vi "Start.vi"(6 "Load FP? (T)":bool=TRUE, 8 "error in (no error)":errorcluster, 9 "Data":string, 10 "Name":string, 11 "VI Reference in":variant) -> (0 "error out":errorcluster, 2 "Generic VI Reference":refnum<vi>, 3 "VI Reference out":variant)   [LabVIEW 2021, in "Thread.lvlib"]
uses:
  Thread.lvlib
  <vilib>/Utility/error.llb/Error Cluster From Error Code.vi
  <vilib>/ErrorRing/Error Ring.xnode
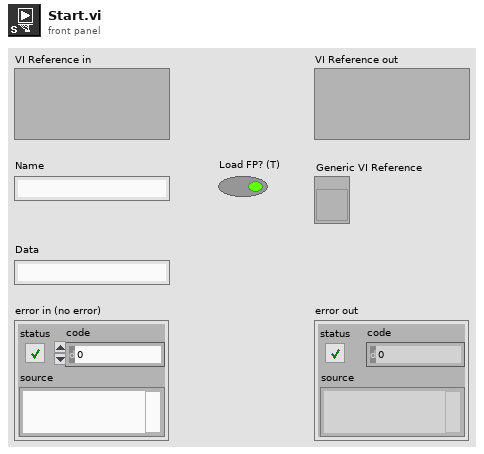
[diagram p1: front panel]
types:
  T1 = enum32{"Invalid", "Standard", "Closed", "Hidden", "Minimized", "Maximized"}
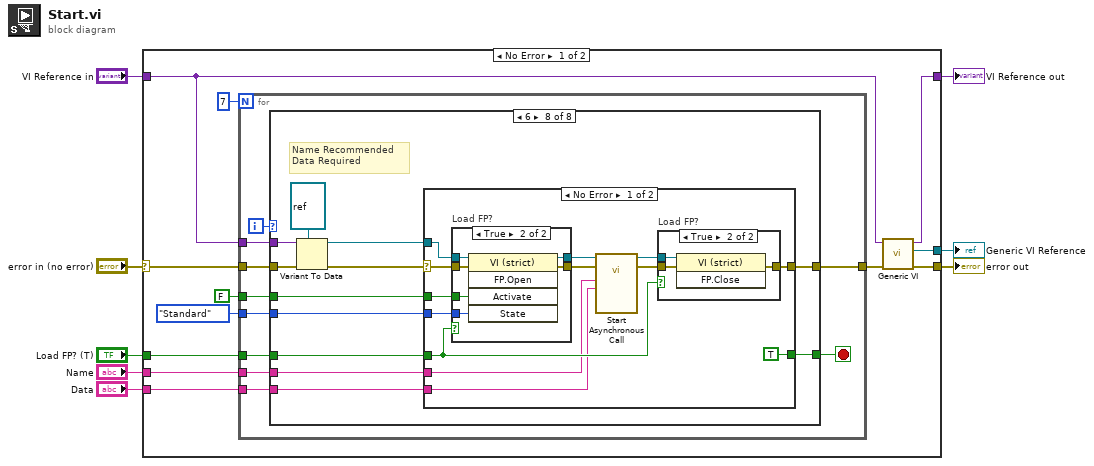
[diagram p0: block diagram]
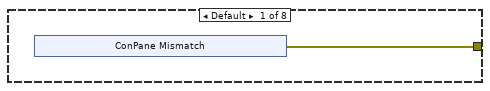
[diagram p2: hidden frame]
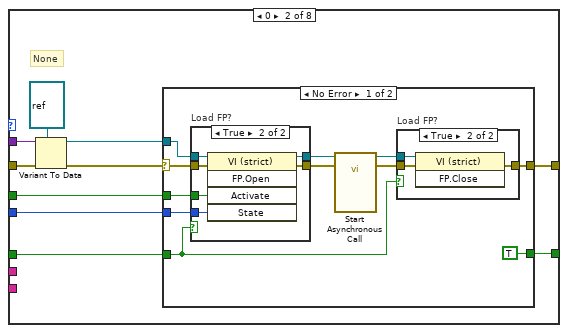
[diagram p3: hidden frame]
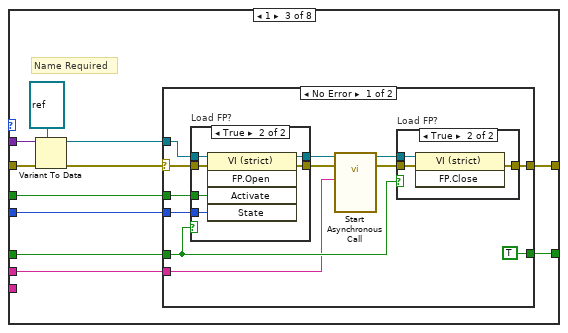
[diagram p7: hidden frame]
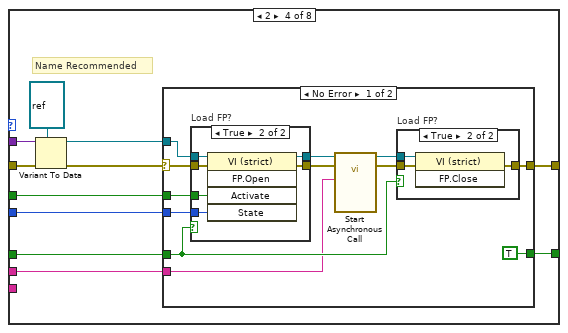
[diagram p11: hidden frame]
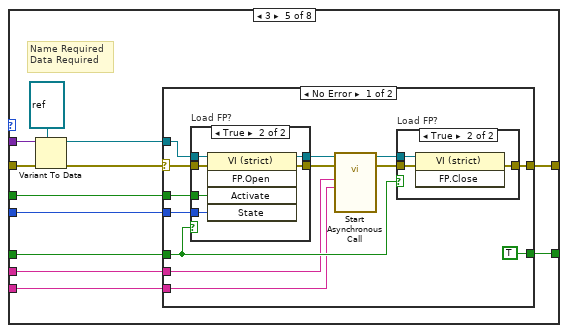
[diagram p15: hidden frame]
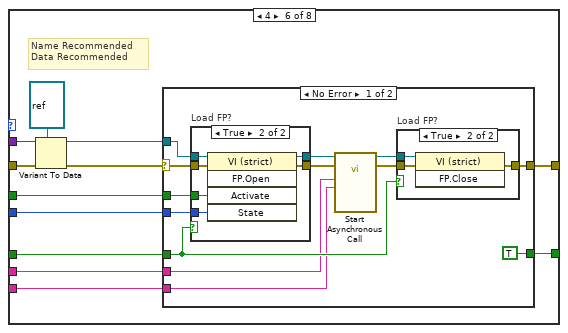
[diagram p19: hidden frame]
diagram:
  n1 = case shown="No Error" "error in (no error)" {
    selector: "error in (no error)" -> [w20 w294]
    tunnel: "VI Reference in" -> [w9 _]
    tunnel: [w12 w294] -> w7
    tunnel: [w10 _] -> w6
    tunnel: [w11 _] -> w5
    tunnel: "Load FP? (T)" -> [w18 _]
    tunnel: "Name" -> [w17 _]
    tunnel: "Data" -> [w16 _]
    frame No Error {
      n2 = for {
        N: 7 -> [_]
        tunnel: w9 -> [w29]
        tunnel: w20 -> [w30]
        tunnel: [w27] -> w13
        tunnel: w18 -> [w26]
        tunnel: w17 -> [w25]
        tunnel: w16 -> [w24]
        tunnel: FALSE ("Activate?") -> [w23]
        tunnel: T1."Standard" ("State") -> [w22]
        i -> [w28]
        stop <- w21 stop-if-true
        n3 = case shown="6" w28 {
          tunnel: w30 -> [_ w45 w80 w116 w153 w191 w229 w267]
          tunnel: w29 -> [_ w43 w78 w114 w151 w189 w227 w265]
          tunnel: [w31 w41 w76 w112 w149 w187 w225 w263] -> w27
          tunnel: w26 -> [_ w39 w75 w111 w148 w186 w224 w262]
          tunnel: w25 -> [_ _ w70 w106 w144 w182 w220 w258]
          tunnel: w24 -> [_ _ _ _ w142 w181 w219 w257]
          tunnel: w23 -> [_ w38 w74 w110 w147 w185 w223 w261]
          tunnel: w22 -> [_ w37 w73 w109 w146 w184 w222 w260]
          tunnel: [_ w36 w72 w108 w145 w183 w221 w259] -> w21
          frame Default {
            n4 = xnode "ConPane Mismatch"() -> ("error out"=w31:errorcluster)
          }
          frame 0 {
            # "None"
            n5 = Variant To Data(error in=w45, type=refnum<vi> refnum ("VI Refnum"), Variant=w43) -> (data=w42:refnum<vi>, error out=w44:errorcluster)
            n6 = case shown="No Error" w44 {
              selector: w44 -> [w56 w69]
              tunnel: w42 -> [w53 _]
              tunnel: [w51 w69] -> w41
              tunnel: w39 -> [w49 _]
              tunnel: w38 -> [w48 _]
              tunnel: w37 -> [w47 _]
              tunnel: [TRUE _] -> w36
              frame No Error {
                n7 = case "Load FP?" shown="True" w49 {
                  tunnel: w56 -> [w62 w68]
                  tunnel: [w62 w67] -> w54
                  tunnel: w53 -> [w61 w66]
                  tunnel: [w61 w65] -> w52
                  tunnel: w48 -> [_ w64]
                  tunnel: w47 -> [_ w63]
                  frame False {
                  }
                  frame True {
                    n8 = invoke class="VI (strict)" method="FP.Open"(reference=w66, error in=w68, "Activate"=w64, "State"=w63) -> (reference out=w65:refnum<vi>, error out=w67:errorcluster)  [unwired: 1 in, 3 out]
                  }
                }
                n9 = call-by-ref "Start Asynchronous Call"(reference=w52, error in=w54) -> (reference out=w50:refnum<vi>, error out=w55:errorcluster)  [unwired: 12 in]
                n10 = case "Load FP?" shown="True" w49 {
                  tunnel: w55 -> [w57 w60]
                  tunnel: [w57 w59] -> w51
                  tunnel: w50 -> [_ w58]
                  frame False {
                  }
                  frame True {
                    n11 = invoke class="VI (strict)" method="FP.Close"(reference=w58, error in=w60) -> (error out=w59:errorcluster)  [unwired: 1 in, 2 out]
                  }
                }
              }
              frame Error {
              }
            }
          }
          frame 1 {
            # "Name Required"
            n12 = Variant To Data(error in=w80, type=refnum<vi> refnum ("VI Refnum"), Variant=w78) -> (data=w77:refnum<vi>, error out=w79:errorcluster)
            n13 = case shown="No Error" w79 {
              selector: w79 -> [w92 w105]
              tunnel: w77 -> [w89 _]
              tunnel: [w87 w105] -> w76
              tunnel: w75 -> [w85 _]
              tunnel: w74 -> [w84 _]
              tunnel: w73 -> [w83 _]
              tunnel: [TRUE _] -> w72
              tunnel: w70 -> [w81 _]
              frame No Error {
                n14 = case "Load FP?" shown="True" w85 {
                  tunnel: w92 -> [w98 w104]
                  tunnel: [w98 w103] -> w90
                  tunnel: w89 -> [w97 w102]
                  tunnel: [w97 w101] -> w88
                  tunnel: w84 -> [_ w100]
                  tunnel: w83 -> [_ w99]
                  frame False {
                  }
                  frame True {
                    n15 = invoke class="VI (strict)" method="FP.Open"(reference=w102, error in=w104, "Activate"=w100, "State"=w99) -> (reference out=w101:refnum<vi>, error out=w103:errorcluster)  [unwired: 1 in, 3 out]
                  }
                }
                n16 = call-by-ref "Start Asynchronous Call"(reference=w88, error in=w90, "Name"=w81) -> (reference out=w86:refnum<vi>, error out=w91:errorcluster)  [unwired: 11 in]
                n17 = case "Load FP?" shown="True" w85 {
                  tunnel: w91 -> [w93 w96]
                  tunnel: [w93 w95] -> w87
                  tunnel: w86 -> [_ w94]
                  frame False {
                  }
                  frame True {
                    n18 = invoke class="VI (strict)" method="FP.Close"(reference=w94, error in=w96) -> (error out=w95:errorcluster)  [unwired: 1 in, 2 out]
                  }
                }
              }
              frame Error {
              }
            }
          }
          frame 2 {
            # "Name Recommended"
            n19 = Variant To Data(error in=w116, type=refnum<vi> refnum ("VI Refnum"), Variant=w114) -> (data=w113:refnum<vi>, error out=w115:errorcluster)
            n20 = case shown="No Error" w115 {
              selector: w115 -> [w128 w141]
              tunnel: w113 -> [w125 _]
              tunnel: [w123 w141] -> w112
              tunnel: w111 -> [w121 _]
              tunnel: w110 -> [w120 _]
              tunnel: w109 -> [w119 _]
              tunnel: [TRUE _] -> w108
              tunnel: w106 -> [w117 _]
              frame No Error {
                n21 = case "Load FP?" shown="True" w121 {
                  tunnel: w128 -> [w134 w140]
                  tunnel: [w134 w139] -> w126
                  tunnel: w125 -> [w133 w138]
                  tunnel: [w133 w137] -> w124
                  tunnel: w120 -> [_ w136]
                  tunnel: w119 -> [_ w135]
                  frame False {
                  }
                  frame True {
                    n22 = invoke class="VI (strict)" method="FP.Open"(reference=w138, error in=w140, "Activate"=w136, "State"=w135) -> (reference out=w137:refnum<vi>, error out=w139:errorcluster)  [unwired: 1 in, 3 out]
                  }
                }
                n23 = call-by-ref "Start Asynchronous Call"(reference=w124, error in=w126, "Name"=w117) -> (reference out=w122:refnum<vi>, error out=w127:errorcluster)  [unwired: 11 in]
                n24 = case "Load FP?" shown="True" w121 {
                  tunnel: w127 -> [w129 w132]
                  tunnel: [w129 w131] -> w123
                  tunnel: w122 -> [_ w130]
                  frame False {
                  }
                  frame True {
                    n25 = invoke class="VI (strict)" method="FP.Close"(reference=w130, error in=w132) -> (error out=w131:errorcluster)  [unwired: 1 in, 2 out]
                  }
                }
              }
              frame Error {
              }
            }
          }
          frame 3 {
            # "Name Required\nData Required"
            n26 = Variant To Data(error in=w153, type=refnum<vi> refnum ("VI Refnum"), Variant=w151) -> (data=w150:refnum<vi>, error out=w152:errorcluster)
            n27 = case shown="No Error" w152 {
              selector: w152 -> [w166 w179]
              tunnel: w150 -> [w163 _]
              tunnel: [w161 w179] -> w149
              tunnel: w148 -> [w159 _]
              tunnel: w147 -> [w158 _]
              tunnel: w146 -> [w157 _]
              tunnel: [TRUE _] -> w145
              tunnel: w144 -> [w155 _]
              tunnel: w142 -> [w154 _]
              frame No Error {
                n28 = case "Load FP?" shown="True" w159 {
                  tunnel: w166 -> [w172 w178]
                  tunnel: [w172 w177] -> w164
                  tunnel: w163 -> [w171 w176]
                  tunnel: [w171 w175] -> w162
                  tunnel: w158 -> [_ w174]
                  tunnel: w157 -> [_ w173]
                  frame False {
                  }
                  frame True {
                    n29 = invoke class="VI (strict)" method="FP.Open"(reference=w176, error in=w178, "Activate"=w174, "State"=w173) -> (reference out=w175:refnum<vi>, error out=w177:errorcluster)  [unwired: 1 in, 3 out]
                  }
                }
                n30 = call-by-ref "Start Asynchronous Call"(reference=w162, error in=w164, "Data"=w154, "Name"=w155) -> (reference out=w160:refnum<vi>, error out=w165:errorcluster)  [unwired: 10 in]
                n31 = case "Load FP?" shown="True" w159 {
                  tunnel: w165 -> [w167 w170]
                  tunnel: [w167 w169] -> w161
                  tunnel: w160 -> [_ w168]
                  frame False {
                  }
                  frame True {
                    n32 = invoke class="VI (strict)" method="FP.Close"(reference=w168, error in=w170) -> (error out=w169:errorcluster)  [unwired: 1 in, 2 out]
                  }
                }
              }
              frame Error {
              }
            }
          }
          frame 4 {
            # "Name Recommended\nData Recommended"
            n33 = Variant To Data(error in=w191, type=refnum<vi> refnum ("VI Refnum"), Variant=w189) -> (data=w188:refnum<vi>, error out=w190:errorcluster)
            n34 = case shown="No Error" w190 {
              selector: w190 -> [w204 w217]
              tunnel: w188 -> [w201 _]
              tunnel: [w199 w217] -> w187
              tunnel: w186 -> [w197 _]
              tunnel: w185 -> [w196 _]
              tunnel: w184 -> [w195 _]
              tunnel: [TRUE _] -> w183
              tunnel: w182 -> [w193 _]
              tunnel: w181 -> [w192 _]
              frame No Error {
                n35 = case "Load FP?" shown="True" w197 {
                  tunnel: w204 -> [w210 w216]
                  tunnel: [w210 w215] -> w202
                  tunnel: w201 -> [w209 w214]
                  tunnel: [w209 w213] -> w200
                  tunnel: w196 -> [_ w212]
                  tunnel: w195 -> [_ w211]
                  frame False {
                  }
                  frame True {
                    n36 = invoke class="VI (strict)" method="FP.Open"(reference=w214, error in=w216, "Activate"=w212, "State"=w211) -> (reference out=w213:refnum<vi>, error out=w215:errorcluster)  [unwired: 1 in, 3 out]
                  }
                }
                n37 = call-by-ref "Start Asynchronous Call"(reference=w200, error in=w202, "Data"=w192, "Name"=w193) -> (reference out=w198:refnum<vi>, error out=w203:errorcluster)  [unwired: 10 in]
                n38 = case "Load FP?" shown="True" w197 {
                  tunnel: w203 -> [w205 w208]
                  tunnel: [w205 w207] -> w199
                  tunnel: w198 -> [_ w206]
                  frame False {
                  }
                  frame True {
                    n39 = invoke class="VI (strict)" method="FP.Close"(reference=w206, error in=w208) -> (error out=w207:errorcluster)  [unwired: 1 in, 2 out]
                  }
                }
              }
              frame Error {
              }
            }
          }
          frame 5 {
            # "Name Required\nData Recommended"
            n40 = Variant To Data(error in=w229, type=refnum<vi> refnum ("VI Refnum"), Variant=w227) -> (data=w226:refnum<vi>, error out=w228:errorcluster)
            n41 = case shown="No Error" w228 {
              selector: w228 -> [w242 w255]
              tunnel: w226 -> [w239 _]
              tunnel: [w237 w255] -> w225
              tunnel: w224 -> [w235 _]
              tunnel: w223 -> [w234 _]
              tunnel: w222 -> [w233 _]
              tunnel: [TRUE _] -> w221
              tunnel: w220 -> [w231 _]
              tunnel: w219 -> [w230 _]
              frame No Error {
                n42 = case "Load FP?" shown="True" w235 {
                  tunnel: w242 -> [w248 w254]
                  tunnel: [w248 w253] -> w240
                  tunnel: w239 -> [w247 w252]
                  tunnel: [w247 w251] -> w238
                  tunnel: w234 -> [_ w250]
                  tunnel: w233 -> [_ w249]
                  frame False {
                  }
                  frame True {
                    n43 = invoke class="VI (strict)" method="FP.Open"(reference=w252, error in=w254, "Activate"=w250, "State"=w249) -> (reference out=w251:refnum<vi>, error out=w253:errorcluster)  [unwired: 1 in, 3 out]
                  }
                }
                n44 = call-by-ref "Start Asynchronous Call"(reference=w238, error in=w240, "Data"=w230, "Name"=w231) -> (reference out=w236:refnum<vi>, error out=w241:errorcluster)  [unwired: 10 in]
                n45 = case "Load FP?" shown="True" w235 {
                  tunnel: w241 -> [w243 w246]
                  tunnel: [w243 w245] -> w237
                  tunnel: w236 -> [_ w244]
                  frame False {
                  }
                  frame True {
                    n46 = invoke class="VI (strict)" method="FP.Close"(reference=w244, error in=w246) -> (error out=w245:errorcluster)  [unwired: 1 in, 2 out]
                  }
                }
              }
              frame Error {
              }
            }
          }
          frame 6 {
            # "Name Recommended\nData Required"
            n47 = Variant To Data(error in=w267, type=refnum<vi> refnum ("VI Refnum"), Variant=w265) -> (data=w264:refnum<vi>, error out=w266:errorcluster)
            n48 = case shown="No Error" w266 {
              selector: w266 -> [w280 w293]
              tunnel: w264 -> [w277 _]
              tunnel: [w275 w293] -> w263
              tunnel: w262 -> [w273 _]
              tunnel: w261 -> [w272 _]
              tunnel: w260 -> [w271 _]
              tunnel: [TRUE _] -> w259
              tunnel: w258 -> [w269 _]
              tunnel: w257 -> [w268 _]
              frame No Error {
                n49 = case "Load FP?" shown="True" w273 {
                  tunnel: w280 -> [w286 w292]
                  tunnel: [w286 w291] -> w278
                  tunnel: w277 -> [w285 w290]
                  tunnel: [w285 w289] -> w276
                  tunnel: w272 -> [_ w288]
                  tunnel: w271 -> [_ w287]
                  frame False {
                  }
                  frame True {
                    n50 = invoke class="VI (strict)" method="FP.Open"(reference=w290, error in=w292, "Activate"=w288, "State"=w287) -> (reference out=w289:refnum<vi>, error out=w291:errorcluster)  [unwired: 1 in, 3 out]
                  }
                }
                n51 = call-by-ref "Start Asynchronous Call"(reference=w276, error in=w278, "Data"=w268, "Name"=w269) -> (reference out=w274:refnum<vi>, error out=w279:errorcluster)  [unwired: 10 in]
                n52 = case "Load FP?" shown="True" w273 {
                  tunnel: w279 -> [w281 w284]
                  tunnel: [w281 w283] -> w275
                  tunnel: w274 -> [_ w282]
                  frame False {
                  }
                  frame True {
                    n53 = invoke class="VI (strict)" method="FP.Close"(reference=w282, error in=w284) -> (error out=w283:errorcluster)  [unwired: 1 in, 2 out]
                  }
                }
              }
              frame Error {
              }
            }
          }
        }
      }
      n54 = call "Generic VI.vi"("error in (no error)"=w13, "VI Reference in"=w9) -> ("error out"=w12:errorcluster, "Generic VI Reference"=w11:refnum<vi>, "VI Reference out"=w10:variant)  [unwired: 7 in]
    }
    frame Error {
    }
  }
  "error out" <- w7
  "Generic VI Reference" <- w5
  "VI Reference out" <- w6
